vi "motorRMX.vi"(12 "error in":errorcluster) -> (14 "error out":errorcluster)   [LabVIEW 2018]
uses:
  <vilib>/DAQmx/read.llb/DAQmx Read (Analog 1D Wfm NChan NSamp).vi
  <vilib>/DAQmx/write.llb/DAQmx Write (Digital 1D Bool NChan 1Samp 1Line).vi
  <vilib>/DAQmx/write.llb/DAQmx Write (Analog 1D DBL NChan 1Samp).vi
  <vilib>/DAQmx/create/channels.llb/DAQmx Create Channel (AI-Voltage-Basic).vi
  <vilib>/DAQmx/configure/timing.llb/DAQmx Timing (Sample Clock).vi
  <vilib>/DAQmx/create/channels.llb/DAQmx Create Channel (DO-Digital Output).vi
  <vilib>/DAQmx/create/channels.llb/DAQmx Create Channel (AO-Voltage-Basic).vi
  <vilib>/DAQmx/miscellaneous.llb/DAQmx Fill In Error Info.vi
  <resource>/objmgr/daqmx.rc
panel:
  in  "Station 4":bool
  in  "Station 3":bool
  in  "Station 2":bool
  in  "Station1":bool
  out "appended array":bool[](array[boolean])
  in  "Cycles":i16
  in  "Cycles":i16
  in  "Cycles":i16
  in  "Cycles":i16
  out "Cycles ran 4":i16
  out "Cycles ran3":i16
  out "Cycles Ran2":i16
  out "Cycles ran 1":i16
  out "Torque ch 4":dbl format="%0.2f"
  out "Torque Ch 3":dbl format="%0.2f"
  out "Torque ch 2":dbl format="%0.2f"
  out "Torque ch 1":dbl format="%0.2f"
  in  "stop":bool
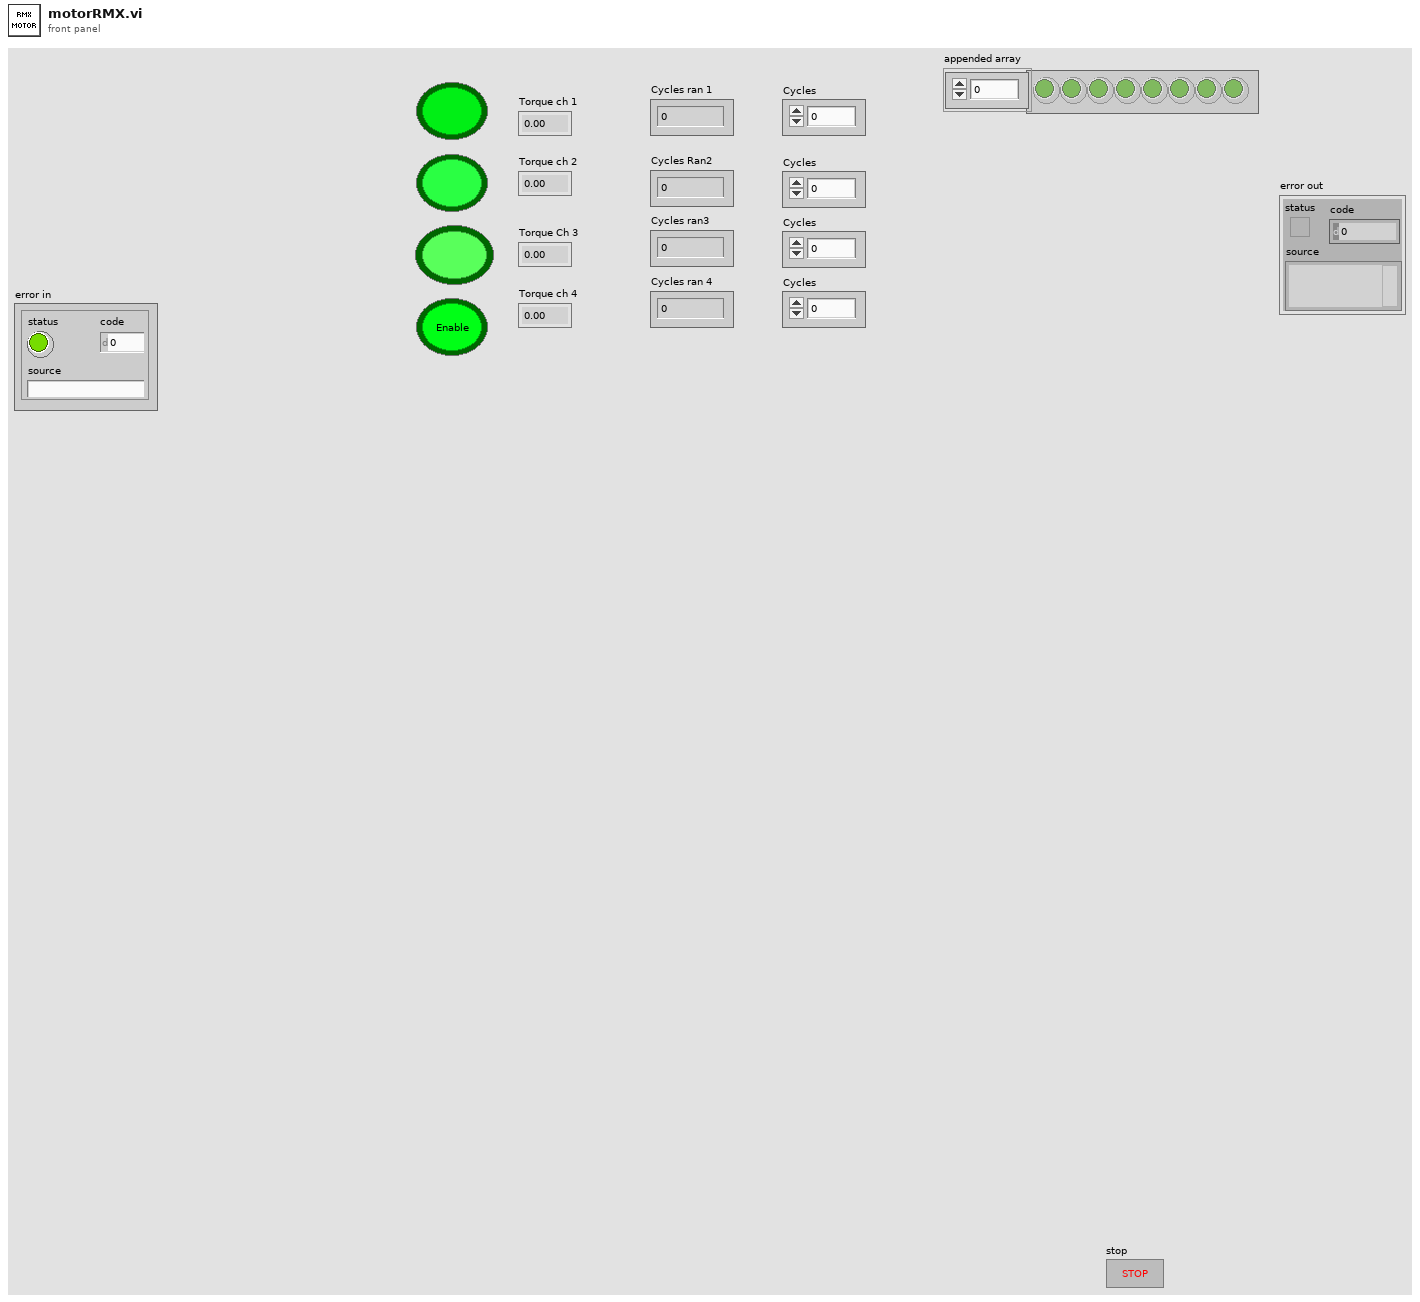
[diagram p1: front panel]
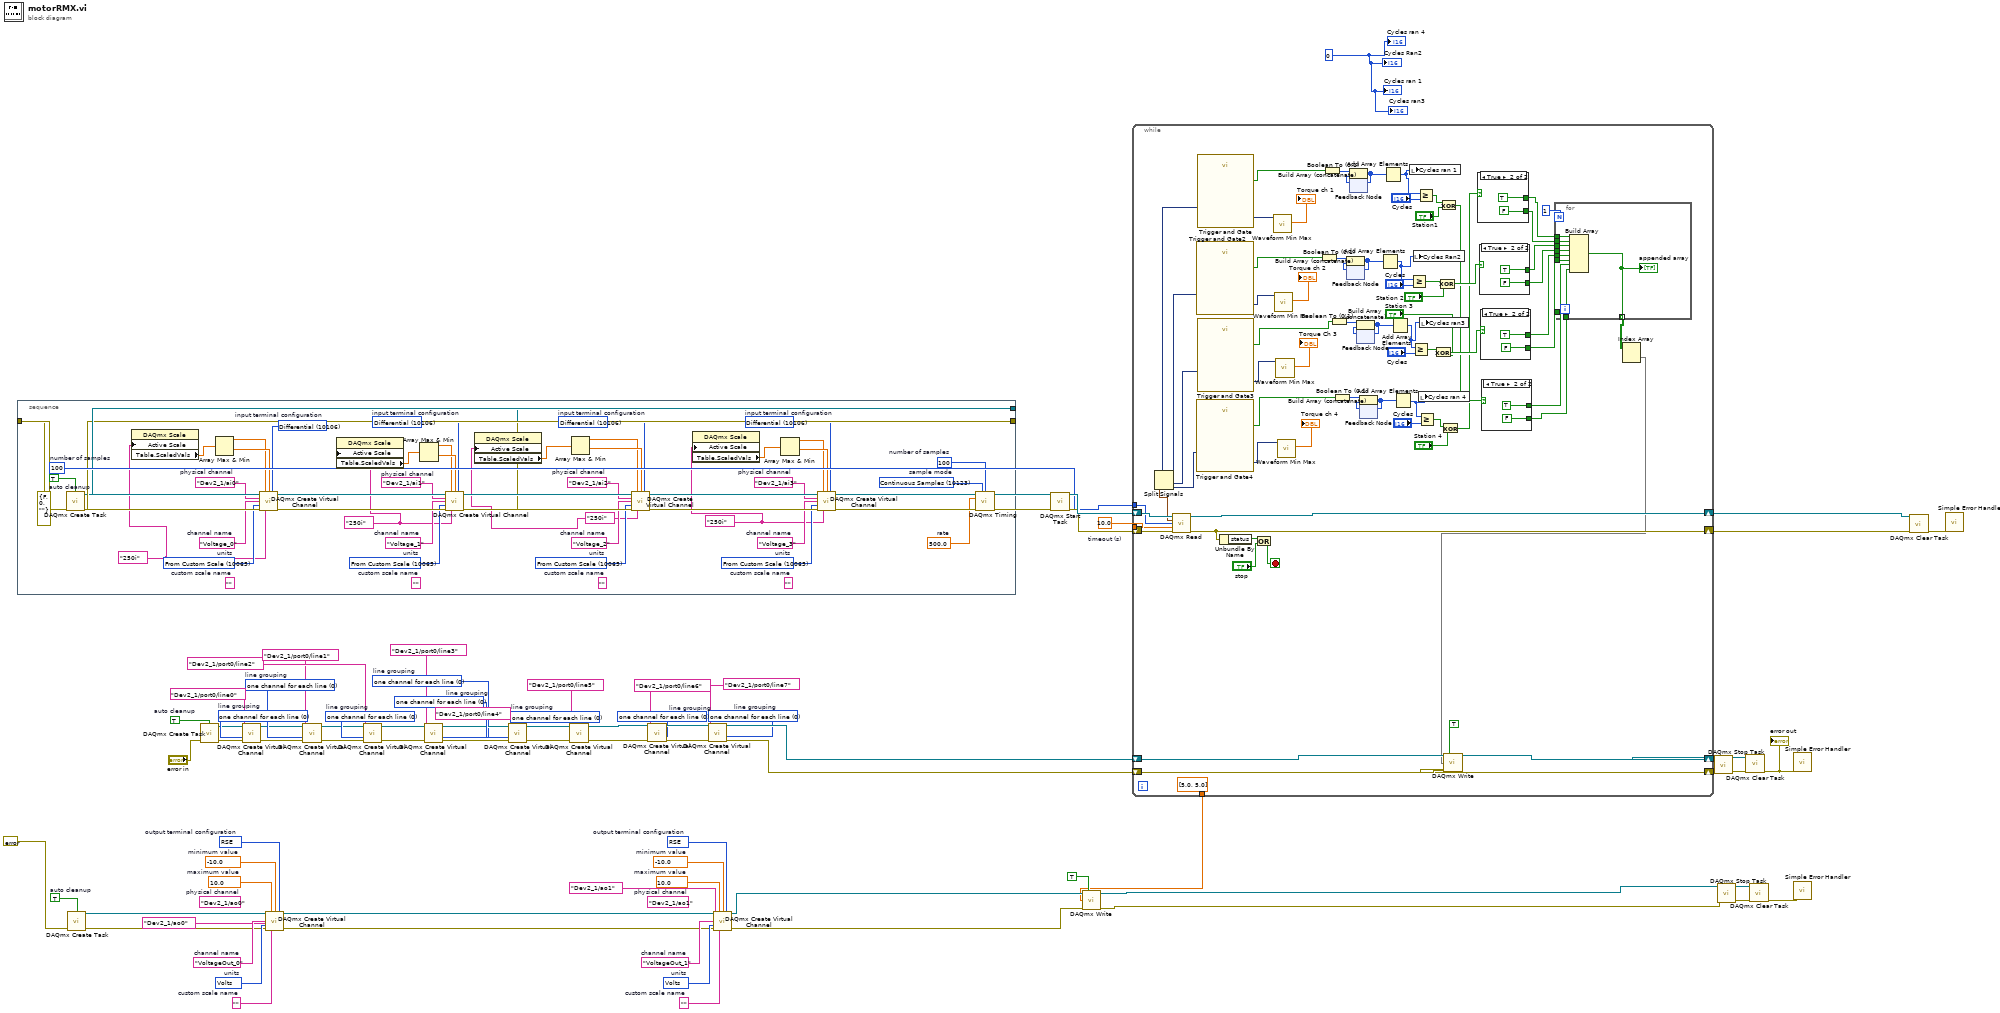
[diagram p0: block diagram]
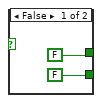
[diagram p2: hidden frame]
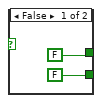
[diagram p3: hidden frame]
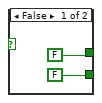
[diagram p4: hidden frame]
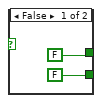
[diagram p5: hidden frame]
diagram:
  w1 = 0
  w8 = 10.0  # timeout (s)
  w15 = 100  # number of samples
  w36 = 10083 items=["Default"=-1, "RSE"=10083, "Differential"=10106, "Pseudodifferential"=12529]  # output terminal configuration
  w35 = 10348 items=["Volts"=10348, "From Custom Scale"=10065]  # units
  w34 = "VoltageOut_1"  # channel name
  w33 = ""  # custom scale name
  w32 = -10.0  # minimum value
  w31 = 10.0  # maximum value
  (unwired) "Dev2_1/ao1"  # physical channel
  w29 = 10083 items=["Default"=-1, "RSE"=10083, "Differential"=10106, "Pseudodifferential"=12529]  # output terminal configuration
  w28 = 10348 items=["Volts"=10348, "From Custom Scale"=10065]  # units
  w27 = "VoltageOut_0"  # channel name
  w25 = ""  # custom scale name
  w24 = -10.0  # minimum value
  w23 = 10.0  # maximum value
  (unwired) "Dev2_1/ao0"  # physical channel
  w21 = TRUE  # auto cleanup
  w78 = 0 items=["one channel for each line", "one channel for all lines"]  # line grouping
  w75 = 0 items=["one channel for each line", "one channel for all lines"]  # line grouping
  w72 = 0 items=["one channel for each line", "one channel for all lines"]  # line grouping
  w69 = 0 items=["one channel for each line", "one channel for all lines"]  # line grouping
  w66 = 0 items=["one channel for each line", "one channel for all lines"]  # line grouping
  w63 = 0 items=["one channel for each line", "one channel for all lines"]  # line grouping
  w60 = 0 items=["one channel for each line", "one channel for all lines"]  # line grouping
  w57 = 0 items=["one channel for each line", "one channel for all lines"]  # line grouping
  w55 = TRUE  # auto cleanup
  n1 = stacked-sequence {
    tunnel: [w126] -> w11
    tunnel: [w125] -> w12
    tunnel: errorcluster {"status"=FALSE, "code"=0, "source"=""} ("error in") -> [w98]
    frame #0 {
      w85 = tag "250i" ("custom scale name 3")
      w89 = tag "250i" ("custom scale name 2")
      w93 = tag "250i" ("custom scale name")
      w97 = tag "250i" ("custom scale name")
      w130 = 10123 items=["Finite Samples"=10178, "Continuous Samples"=10123, "Hardware Timed Single Point"=12522]  # sample mode
      w129 = 100  # number of samples
      w128 = 500.0  # rate
      w124 = 10106 items=["default"=-1, "RSE"=10083, "NRSE"=10078, "Differential"=10106, "Pseudodifferential"=12529]  # input terminal configuration
      w123 = 10065 items=["Volts"=10348, "From Custom Scale"=10065]  # units
      w122 = "Voltage_3"  # channel name
      (unwired) ""  # custom scale name
      w120 = "Dev2_1/ai3"  # physical channel
      w118 = 10106 items=["default"=-1, "RSE"=10083, "NRSE"=10078, "Differential"=10106, "Pseudodifferential"=12529]  # input terminal configuration
      w117 = 10065 items=["Volts"=10348, "From Custom Scale"=10065]  # units
      w116 = "Voltage_2"  # channel name
      (unwired) ""  # custom scale name
      w114 = "Dev2_1/ai2"  # physical channel
      w112 = 10106 items=["default"=-1, "RSE"=10083, "NRSE"=10078, "Differential"=10106, "Pseudodifferential"=12529]  # input terminal configuration
      w111 = 10065 items=["Volts"=10348, "From Custom Scale"=10065]  # units
      w110 = "Voltage_1"  # channel name
      (unwired) ""  # custom scale name
      w108 = "Dev2_1/ai1"  # physical channel
      w106 = 10106 items=["default"=-1, "RSE"=10083, "NRSE"=10078, "Differential"=10106, "Pseudodifferential"=12529]  # input terminal configuration
      w105 = 10065 items=["Volts"=10348, "From Custom Scale"=10065]  # units
      w104 = "Voltage_0"  # channel name
      (unwired) ""  # custom scale name
      w102 = "Dev2_1/ai0"  # physical channel
      w100 = TRUE  # auto cleanup
      n2 = call <vilib>:"DAQmx Create Task.vi"("auto cleanup"=w100, "error in"=w98) -> ("task out"=w101:refnum<k21>, "error out"=w99:errorcluster)  [unwired: 12 in]
      n3 = property class="DAQmx Scale"("Active Scale"=w97) -> ("Table.ScaledVals"=w96:dbl[])  [unwired: 2 in, 2 out]
      n4 = Array Max & Min(array=w96) -> (max value=w94:dbl, min value=w95:dbl)  [unwired: 2 out]
      n5 = call-poly <vilib>:"DAQmx Create Virtual Channel.vi"("task in"=w101, "maximum value"=w94, "minimum value"=w95, "input terminal configuration"=w106, "physical channels"=w102, "name to assign"=w104, "units"=w105, "error in"=w99, "custom scale name"=w97) -> ("task out"=w107:refnum<k21>, "error out"=w103:errorcluster)  [unwired: 5 in]
      n6 = property class="DAQmx Scale"("Active Scale"=w93) -> ("Table.ScaledVals"=w92:dbl[])  [unwired: 2 in, 2 out]
      n7 = Array Max & Min(array=w92) -> (max value=w90:dbl, min value=w91:dbl)  [unwired: 2 out]
      n8 = call-poly <vilib>:"DAQmx Create Virtual Channel.vi"("task in"=w107, "maximum value"=w90, "minimum value"=w91, "input terminal configuration"=w112, "physical channels"=w108, "name to assign"=w110, "units"=w111, "error in"=w103, "custom scale name"=w93) -> ("task out"=w113:refnum<k21>, "error out"=w109:errorcluster)  [unwired: 5 in]
      n9 = property class="DAQmx Scale"("Active Scale"=w89) -> ("Table.ScaledVals"=w88:dbl[])  [unwired: 2 in, 2 out]
      n10 = Array Max & Min(array=w88) -> (max value=w86:dbl, min value=w87:dbl)  [unwired: 2 out]
      n11 = call-poly <vilib>:"DAQmx Create Virtual Channel.vi"("task in"=w113, "maximum value"=w86, "minimum value"=w87, "input terminal configuration"=w118, "physical channels"=w114, "name to assign"=w116, "units"=w117, "error in"=w109, "custom scale name"=w89) -> ("task out"=w119:refnum<k21>, "error out"=w115:errorcluster)  [unwired: 5 in]
      n12 = property class="DAQmx Scale"("Active Scale"=w85) -> ("Table.ScaledVals"=w84:dbl[])  [unwired: 2 in, 2 out]
      n13 = Array Max & Min(array=w84) -> (max value=w82:dbl, min value=w83:dbl)  [unwired: 2 out]
      n14 = call-poly <vilib>:"DAQmx Create Virtual Channel.vi"("task in"=w119, "maximum value"=w82, "minimum value"=w83, "input terminal configuration"=w124, "physical channels"=w120, "name to assign"=w122, "units"=w123, "error in"=w115, "custom scale name"=w85) -> ("task out"=w127:refnum<k21>, "error out"=w121:errorcluster)  [unwired: 5 in]
      n15 = call-poly <vilib>:"DAQmx Timing.vi"("task/channels in"=w127, "sample mode"=w130, "samples per channel"=w129, "rate"=w128, "error in"=w121) -> ("task out"=w125:refnum<k21>, "error out"=w126:errorcluster)  [unwired: 9 in]
    }
  }
  n16 = call <vilib>:"DAQmx Create Task.vi"("auto cleanup"=w21, "error in"=errorcluster {"status"=FALSE, "code"=0, "source"=""}) -> ("task out"=w22:refnum<k21>, "error out"=w20:errorcluster)  [unwired: 12 in]
  n17 = call <vilib>:"DAQmx Create Task.vi"("auto cleanup"=w55, "error in"="error in") -> ("task out"=w56:refnum<k21>, "error out"=w54:errorcluster)  [unwired: 12 in]
  n18 = call-poly <vilib>:"DAQmx Create Virtual Channel.vi"("task in"=w56, "lines"=tag "Dev2_1/port0/line0" ("lines 1"), "line grouping"=w57, "error in"=w54) -> ("task out"=w59:refnum<k21>, "error out"=w58:errorcluster)  [unwired: 10 in]
  n19 = call-poly <vilib>:"DAQmx Create Virtual Channel.vi"("task in"=w22, "maximum value"=w23, "minimum value"=w24, "output terminal configuration"=w29, "physical channels"=tag "Dev2_1/ao0", "name to assign"=w27, "units"=w28, "error in"=w20, "custom scale name"=w25) -> ("task out"=w30:refnum<k21>, "error out"=w26:errorcluster)  [unwired: 5 in]
  n20 = call-poly <vilib>:"DAQmx Create Virtual Channel.vi"("task in"=w59, "lines"=tag "Dev2_1/port0/line1" ("lines 2"), "line grouping"=w60, "error in"=w58) -> ("task out"=w62:refnum<k21>, "error out"=w61:errorcluster)  [unwired: 10 in]
  n21 = call-poly <vilib>:"DAQmx Create Virtual Channel.vi"("task in"=w62, "lines"=tag "Dev2_1/port0/line2" ("lines 3"), "line grouping"=w63, "error in"=w61) -> ("task out"=w65:refnum<k21>, "error out"=w64:errorcluster)  [unwired: 10 in]
  n22 = call-poly <vilib>:"DAQmx Create Virtual Channel.vi"("task in"=w65, "lines"=tag "Dev2_1/port0/line3" ("lines4"), "line grouping"=w66, "error in"=w64) -> ("task out"=w68:refnum<k21>, "error out"=w67:errorcluster)  [unwired: 10 in]
  n23 = call-poly <vilib>:"DAQmx Create Virtual Channel.vi"("task in"=w68, "lines"=tag "Dev2_1/port0/line4" ("lines 5"), "line grouping"=w69, "error in"=w67) -> ("task out"=w71:refnum<k21>, "error out"=w70:errorcluster)  [unwired: 10 in]
  n24 = call-poly <vilib>:"DAQmx Create Virtual Channel.vi"("task in"=w71, "lines"=tag "Dev2_1/port0/line5" ("lines 6"), "line grouping"=w72, "error in"=w70) -> ("task out"=w74:refnum<k21>, "error out"=w73:errorcluster)  [unwired: 10 in]
  n25 = call-poly <vilib>:"DAQmx Create Virtual Channel.vi"("task in"=w74, "lines"=tag "Dev2_1/port0/line6" ("lines 7"), "line grouping"=w75, "error in"=w73) -> ("task out"=w77:refnum<k21>, "error out"=w76:errorcluster)  [unwired: 10 in]
  n26 = call-poly <vilib>:"DAQmx Create Virtual Channel.vi"("task in"=w77, "lines"=tag "Dev2_1/port0/line7" ("lines 8"), "line grouping"=w78, "error in"=w76) -> ("task out"=w81:refnum<k21>, "error out"=w80:errorcluster)  [unwired: 10 in]
  n27 = call-poly <vilib>:"DAQmx Create Virtual Channel.vi"("task in"=w30, "maximum value"=w31, "minimum value"=w32, "output terminal configuration"=w36, "physical channels"=tag "Dev2_1/ao1" ("physical channels 2"), "name to assign"=w34, "units"=w35, "error in"=w26, "custom scale name"=w33) -> ("task out"=w7:refnum<k21>, "error out"=w5:errorcluster)  [unwired: 5 in]
  n28 = call <vilib>:"DAQmx Start Task.vi"("task/channels in"=w12, "error in"=w11) -> ("task out"=w17:refnum<k21>, "error out"=w16:errorcluster)  [unwired: 12 in]
  n29 = while {
    tunnel: w15 -> [w199]
    tunnel: w8 -> [w194]
    shift-right: [w203] -> w45
    shift-left: w81 -> [w205]
    shift-right: [w202] -> w44
    shift-left: w80 -> [w204]
    shift-right: [w197] -> w13
    shift-left: w17 -> [w201]
    shift-right: [w198] -> w14
    shift-left: w16 -> [w200]
    tunnel: [dbl[] [5.0, 5.0] ("Speed")] -> w2
    stop <- w191 stop-if-true
    n30 = call-poly <vilib>:"DAQmx Read.vi"("task/channels in"=w201, "number of samples per channel"=w199, "timeout"=w194, "error in"=w200) -> ("task out"=w197:refnum<k21>, "data"=w193:waveform(dbl)[], "error out"=w198:errorcluster)  [unwired: 9 in]
    n31 = Split Signals(w193) -> (w189:dynamicdata, w188:dynamicdata, w187:dynamicdata, w186:dynamicdata)  [unwired: 4 in]
    n32 = call "Trigger and Gate2"("Signals"=w188) -> ("Triggered Signals"=w184:dynamicdata, "Data Available"=w170:bool)  [unwired: 7 in, 2 out]
    n33 = call "Trigger and Gate4"("Signals"=w186) -> ("Triggered Signals"=w182:dynamicdata, "Data Available"=w163:bool)  [unwired: 7 in, 2 out]
    n34 = call "Trigger and Gate"("Signals"=w189) -> ("Triggered Signals"=w185:dynamicdata, "Data Available"=w177:bool)  [unwired: 7 in, 2 out]
    n35 = call "Trigger and Gate3"("Signals"=w187) -> ("Triggered Signals"=w183:dynamicdata, "Data Available"=w164:bool)  [unwired: 7 in, 2 out]
    n36 = Unbundle By Name(w198) -> ("status"=w196:bool)
    n37 = Or(x=w196, y="stop") -> (x .or. y?=w191:bool)
    n38 = call <vilib>:"Waveform Min Max.vi"("waveform in"=w185) -> ("Y max"=→"Torque ch 1":dbl)  [unwired: 5 in, 5 out]
    n39 = call <vilib>:"Waveform Min Max.vi"("waveform in"=w184) -> ("Y max"=→"Torque ch 2":dbl)  [unwired: 5 in, 5 out]
    n40 = call <vilib>:"Waveform Min Max.vi"("waveform in"=w183) -> ("Y max"=→"Torque Ch 3":dbl)  [unwired: 5 in, 5 out]
    n41 = call <vilib>:"Waveform Min Max.vi"("waveform in"=w182) -> ("Y max"=→"Torque ch 4":dbl)  [unwired: 5 in, 5 out]
    n42 = Boolean To (0,1)(Boolean=w170) -> (0, 1=w171:i16)
    n43 = Boolean To (0,1)(Boolean=w177) -> (0, 1=w176:i16)
    n44 = Boolean To (0,1)(Boolean=w164) -> (0, 1=w169:i16)
    n45 = Boolean To (0,1)(Boolean=w163) -> (0, 1=w165:i16)
    n46 = feedback #1() -> (w172:i16[])  [unwired: 1 in]
    n47 = Build Array (concatenate)(w171, w172) -> (w173:i16[])
    n48 = feedback-in #1(w173) -> ()
    n49 = feedback #2() -> (w175:i16[])  [unwired: 1 in]
    n50 = Build Array (concatenate)(w176, w175) -> (w174:i16[])
    n51 = feedback-in #2(w174) -> ()
    n52 = feedback #3() -> (w168:i16[])  [unwired: 1 in]
    n53 = Build Array (concatenate)(w169, w168) -> (w160:i16[])
    n54 = feedback-in #3(w160) -> ()
    n55 = feedback #4() -> (w166:i16[])  [unwired: 1 in]
    n56 = Build Array (concatenate)(w165, w166) -> (w167:i16[])
    n57 = feedback-in #4(w167) -> ()
    n58 = Add Array Elements(numeric array=w173) -> (sum=w133:i16)
    n59 = Add Array Elements(numeric array=w174) -> (sum=w134:i16)
    n60 = Add Array Elements(numeric array=w160) -> (sum=w132:i16)
    n61 = Add Array Elements(numeric array=w167) -> (sum=w131:i16)
    n62 = local write "Cycles ran 1"(w134) -> ()
    n63 = Greater Or Equal?(x=w133, y="Cycles") -> (x >= y?=w148:bool)
    n64 = Greater Or Equal?(x=w132, y="Cycles") -> (x >= y?=w145:bool)
    n65 = local write "Cycles Ran2"(w133) -> ()
    n66 = Greater Or Equal?(x=w134, y="Cycles") -> (x >= y?=w149:bool)
    n67 = Greater Or Equal?(x=w131, y="Cycles") -> (x >= y?=w142:bool)
    n68 = local write "Cycles ran 4"(w131) -> ()
    n69 = local write "Cycles ran3"(w132) -> ()
    n70 = Exclusive Or(1:"Station 3", 2:w145) -> (0:w144:bool)
    n71 = Exclusive Or(1:"Station 2", 2:w148) -> (0:w147:bool)
    n72 = Exclusive Or(1:"Station1", 2:w149) -> (0:w136:bool)
    n73 = Exclusive Or(1:"Station 4", 2:w142) -> (0:w135:bool)
    n74 = case shown="True" w135 {
      tunnel: [FALSE TRUE] -> w150
      tunnel: [FALSE FALSE] -> w151
      frame False {
      }
      frame True {
      }
    }
    n75 = case shown="True" w147 {
      tunnel: [FALSE TRUE] -> w152
      tunnel: [FALSE FALSE] -> w153
      frame False {
      }
      frame True {
      }
    }
    n76 = case shown="True" w144 {
      tunnel: [FALSE TRUE] -> w154
      tunnel: [FALSE FALSE] -> w155
      frame False {
      }
      frame True {
      }
    }
    n77 = case shown="True" w136 {
      tunnel: [FALSE TRUE] -> w156
      tunnel: [FALSE FALSE] -> w157
      frame False {
      }
      frame True {
      }
    }
    n78 = for {
      N: 1 -> [_]
      tunnel: w157 -> [w226]
      tunnel: w156 -> [w225]
      tunnel: w155 -> [w224]
      tunnel: w154 -> [w223]
      tunnel: w153 -> [w222]
      tunnel: w152 -> [w221]
      tunnel: w151 -> [w220]
      tunnel: w150 -> [w219]
      tunnel: [w218] -> w138 mode=indexing
      n79 = Build Array(w219, w220, w221, w222, w223, w224, w225, w226) -> (w218:bool[])
      "appended array" <- w218
    }
    n80 = Index Array(array=w138) -> (element=w137:bool[])  [unwired: 2 in]
    n81 = call-poly <vilib>:"DAQmx Write.vi"("task/channels in"=w205, "auto start"=TRUE, "data"=w137, "error in"=w204) -> ("task out"=w203:refnum<k21>, "error out"=w202:errorcluster)  [unwired: 9 in, 1 out]
  }
  n82 = call-poly <vilib>:"DAQmx Write.vi"("task/channels in"=w7, "auto start"=TRUE, "data"=w2, "error in"=w5) -> ("task out"=w4:refnum<k21>, "error out"=w3:errorcluster)  [unwired: 9 in, 1 out]
  n83 = call <vilib>:"DAQmx Stop Task.vi"("task/channels in"=w45, "error in"=w44) -> ("task out"=w43:refnum<k21>, "error out"=w42:errorcluster)  [unwired: 12 in]
  n84 = call <vilib>:"DAQmx Stop Task.vi"("task/channels in"=w4, "error in"=w3) -> ("task out"=w41:refnum<k21>, "error out"=w40:errorcluster)  [unwired: 12 in]
  n85 = call <vilib>:"DAQmx Clear Task.vi"("task in"=w43, "error in"=w42) -> ("error out"=w39:errorcluster)  [unwired: 13 in]
  "error out" <- w39
  n86 = call <vilib>:"DAQmx Clear Task.vi"("task in"=w41, "error in"=w40) -> ("error out"=w38:errorcluster)  [unwired: 13 in]
  n87 = call <vilib>:"Simple Error Handler.vi"("error in (no error)"=w39) -> ()  [unwired: 4 in, 5 out]
  n88 = call <vilib>:"Simple Error Handler.vi"("error in (no error)"=w38) -> ()  [unwired: 4 in, 5 out]
  n89 = call <vilib>:"DAQmx Clear Task.vi"("task in"=w13, "error in"=w14) -> ("error out"=w9:errorcluster)  [unwired: 13 in]
  n90 = call <vilib>:"Simple Error Handler.vi"("error in (no error)"=w9) -> ()  [unwired: 4 in, 5 out]
  "Cycles ran 1" <- w1
  "Cycles Ran2" <- w1
  "Cycles ran3" <- w1
  "Cycles ran 4" <- w1
